vi "Intake Teleop Handler.vi"() -> ()   [LabVIEW 2025]
uses:
  <vilib>/Rock Robotics/WPI/Joystick/XBox Buttons Indexer.ctl
  <vilib>/Rock Robotics/WPI/Joystick/XBox Axes Indexer.ctl
  34870aaf-5915-4c9e-b01e-bd8868b2fd9e.vi
  <vilib>/Rock Robotics/WPI/Utilities/WPI_GetSetVariantRefNum.vi
panel:
  in  "Upward Power":dbl=-0.30000000000000004
  in  "Downward Power":dbl=0.15
  in  "Intake Speed":dbl=0.75
  # "todo\nshooter keeps running 3sec after intaking stops\ndefalt shooter speed when camera sees nothing"
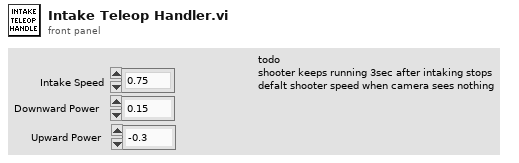
[diagram p1: front panel]
types:
  T1 = typedef "XBox Buttons Indexer.ctl" = enum16{"A", "B", "X", "Y", "Left Bumper", "Right Bumper", "Back", "Start", "Left Joystick", "Right Joystick"}
  T2 = typedef "XBox Axes Indexer.ctl" = enum16{"Left X", "Left Y", "Left Trigger", "Right Trigger", "Right X", "Right Y"}
  T3 = typedef "WPI_JoystickDevRef.ctl" = cluster{"Device":T4}
  T4 = typedef "WPI_JoystickDeviceEnum.ctl" = enum16{"USB 0", "USB 1", "USB 2", "USB 3", "USB 4", "USB 5"}
  T5 = typedef "WPI_MotorControlDeviceRef.ctl" = cluster{"DeviceStatus":errorcluster, "Type":T6, "PWM":cluster{"PWM Channel":T7, "DeadBand":T8}, "CAN":cluster{"Device Number":u8, "SetOutput VI Ref":variant, "GetOutput VI Ref":variant, "Enable VI Ref":variant, "Disable VI Ref":variant, "Data":variant}, "Invert":bool, "DIO PWM":cluster{"PWM \"Enable\" Channel":T7, "DIOChannel":T9, "PWM Rate":dbl}}
  T6 = typedef "WPI_MotorControlType.ctl" = enum16{"PWM", "CAN", "DIO PWM"}
  T7 = typedef "FPGA_DIOPWMChannel.ctl" = enum8{"PWM 0", "PWM 1", "PWM 2", "PWM 3", "PWM 4", "PWM 5", "PWM 6", "PWM 7", "PWM 8", "PWM 9", "PWM MXP 0", "PWM MXP 1", "PWM MXP 2", "PWM MXP 3", "PWM MXP 4", "PWM MXP 5", "PWM MXP 6", "PWM MXP 7", "PWM MXP 8", "PWM MXP 9", "Invalid"}
  T8 = typedef "WPI_PWMDeadband.ctl" = cluster{"Name":string, "maxPositivePwm":i32, "minPositivePwm":i32, "centerPwm":i32, "maxNegativePwm":i32, "minNegativePwm":i32, "angularRange":u16}
  T9 = typedef "FPGA_DIOChannel.ctl" = enum8{"DIO 0", "DIO 1", "DIO 2", "DIO 3", "DIO 4", "DIO 5", "DIO 6", "DIO 7", "DIO 8", "DIO 9", "DIO MXP 0", "DIO MXP 1", "DIO MXP 2", "DIO MXP 3", "DIO MXP 4", "DIO MXP 5", "DIO MXP 6", "DIO MXP 7", "DIO MXP 8", "DIO MXP 9", "DIO MXP 10", "DIO MXP 11", "DIO MXP 12", "DIO MXP 13", "DIO MXP 14", "DIO MXP 15", "SPI Port CS1", "SPI Port CS2", "SPI Port CS3", "SPI Port MISO", "SPI Port MOSI", "Invalid"}
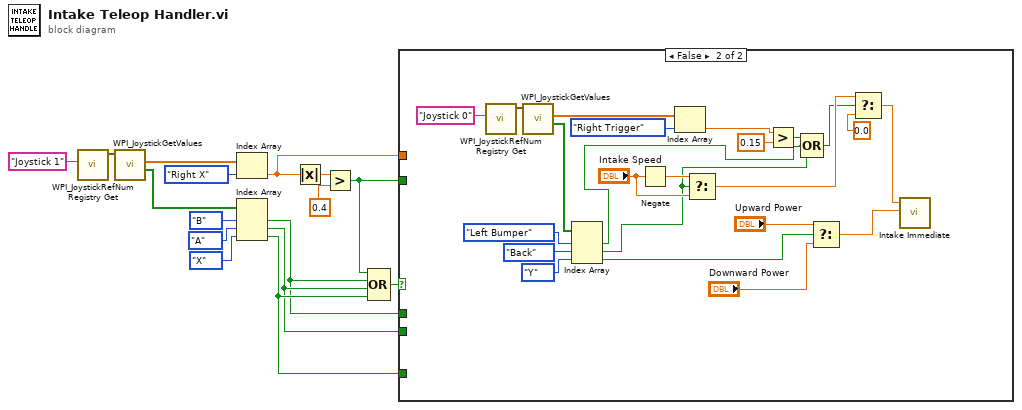
[diagram p0: block diagram]
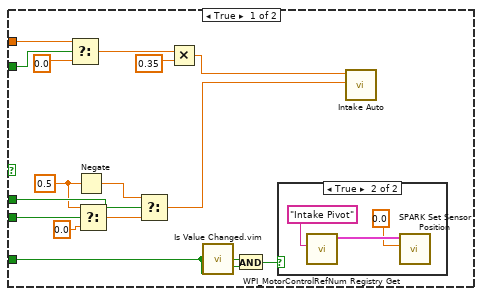
[diagram p2: hidden frame]
diagram:
  n1 = call <vilib>:"WPI_JoystickRefNum Registry Get.vi"("refnum name"="Joystick 1") -> ("JoystickDevRef"=w15:T3)  [unwired: 1 in, 9 out]
  n2 = call <vilib>:"WPI_JoystickGetValues.vi"("JoystickDevRef"=w15) -> ("Buttons"=w11:bool[], "Axes"=w10:dbl[])  [unwired: 6 in, 3 out]
  n3 = Index Array(array=w10, index=XBox_Axes_Indexer."Right X" ("XBox Axes")) -> (element=w8:dbl)
  n4 = Index Array(array=w11, index #1=XBox_Buttons_Indexer."B" ("XBox Buttons"), index #2=XBox_Buttons_Indexer."A" ("XBox Buttons"), index #3=XBox_Buttons_Indexer."X" ("XBox Buttons")) -> (element #1=w2:bool, element #2=w3:bool, element #3=w4:bool)
  n5 = Absolute Value(x=w8) -> (abs(x)=w9:dbl)
  n6 = Greater?(x=w9, y=0.4) -> (0:w1:bool)
  n7 = Compound Arithmetic op=OR(w1, w2, w3, w4) -> (w5:bool)
  n8 = case shown="False" w5 {
    tunnel: w8 -> [w20 _]
    tunnel: w4 -> [w24 _]
    tunnel: w3 -> [w31 _]
    tunnel: w2 -> [w30 _]
    tunnel: w1 -> [w21 _]
    frame True {
      w29 = 0.5 ("t")
      n9 = Select(t=w20, s=w21, f=0.0) -> (s? t:f=w18:dbl)
      n10 = Negate(x=w29) -> (-x=w28:dbl)
      n11 = Select(t=w29, s=w31, f=0.0) -> (s? t:f=w32:dbl)
      n12 = Select(t=w28, s=w30, f=w32) -> (s? t:f=w22:dbl)
      n13 = Multiply(x=w18, y=0.35) -> (x*y=w17:dbl)
      n14 = call "Is Value Changed.vim"("value"=w24) -> ("changed or first call?"=w25:bool)
      n15 = And(x=w25, y=w24) -> (x .and. y?=w23:bool)
      n16 = case shown="True" w23 {
        frame False {
        }
        frame True {
          n17 = call <vilib>:"WPI_MotorControlRefNum Registry Get.vi"("refnum name"="Intake Pivot") -> ("MotorControlDevRef"=w34:T5)  [unwired: 9 in, 1 out]
          n18 = call <vilib>:"SPARK Set Sensor Position.vi"("Position"=0.0, "MotorControlDeviceRef"=w34) -> ()  [unwired: 8 in, 2 out]
        }
      }
      n19 = call "Intake Auto.vi"("Intake Roller Speed"=w22, "Intake Pivot Speed"=w17) -> ()  [unwired: 9 in, 1 out]
    }
    frame False {
      n20 = call <vilib>:"WPI_JoystickRefNum Registry Get.vi"("refnum name"="Joystick 0") -> ("JoystickDevRef"=w57:T3)  [unwired: 1 in, 9 out]
      n21 = call <vilib>:"WPI_JoystickGetValues.vi"("JoystickDevRef"=w57) -> ("Buttons"=w53:bool[], "Axes"=w56:dbl[])  [unwired: 6 in, 3 out]
      n22 = Index Array(array=w53, index #1=XBox_Buttons_Indexer."Left Bumper" ("XBox Buttons"), index #2=XBox_Buttons_Indexer."Back" ("XBox Buttons"), index #3=XBox_Buttons_Indexer."Y" ("XBox Buttons")) -> (element #1=w38:bool, element #2=w37:bool, element #3=w36:bool)
      n23 = Negate(x="Intake Speed") -> (-x=w44:dbl)
      n24 = Index Array(array=w56, index=XBox_Axes_Indexer."Right Trigger" ("XBox Axes")) -> (element=w54:dbl)
      n25 = Select(t=w44, s=w37, f="Intake Speed") -> (s? t:f=w41:dbl)
      n26 = Greater?(x=w54, y=0.15) -> (0:w40:bool)
      n27 = Compound Arithmetic op=OR(w40, w38, w37) -> (w39:bool)
      n28 = Select(t="Upward Power", s=w36, f="Downward Power") -> (s? t:f=w51:dbl)
      n29 = Select(t=w41, s=w39, f=0.0) -> (s? t:f=w50:dbl)
      n30 = call "Intake Immediate.vi"("Intake Pivot Speed"=w51, "Intake Roller Speed"=w50) -> ()  [unwired: 9 in, 1 out]
    }
  }
